vi "自动调阀测试.vi"(8 "error in (no error)":errorcluster caption="错误输入（无错误）") -> (0 "error out":errorcluster caption="错误输出")   [LabVIEW 2015]
doc: "该连续测量范例项目在队列消息处理器模板的基础上实现。\n\n事件处理循环负责按用户界面操作生成对应的消息。\n\n消息处理循环负责对事件处理循环或其他消息生成的消息进行处理。其中还包括用于采集和记录消息处理循环的子VI，以及用于更新图表的循环。"
uses:
  Acquisition/Acquisition.lvlib
  Logging/Logging.lvlib
  support/User Event - Stop/User Event - Stop.lvlib
  support/Message Queue/Message Queue.lvlib
  support/Message Queue/Enqueue Message (Single).vi
  controls/UI Data.ctl
  Measure Type.ctl
  controls/ValueUI Data.ctl
  Action/Action.lvlib
panel:
  out "已完成工序":string
  out "XY Graph":cluster{"Y":dbl[], "Y":dbl[]}[](graph) caption="扭矩VS油压"
  out "XY Graph 2":cluster{"Y":dbl[], "Y":dbl[]}[](graph) caption="角度VS油压"
  out "XY Graph 3":cluster{"Y":dbl[], "Y":dbl[]}[](graph) caption="角度VS扭矩"
  in  "扭杆紧/松":bool
  in  "方向机供油":bool
  in  "夹紧/松阀齿":bool
  in  "夹紧/松阀总":bool
  in  "PLC动作3 5":bool
  in  "PLC动作3 4":bool
  in  "PLC动作3 3":bool
  in  "PLC动作3 2":bool
  in  "PLC动作设置":bool
  in  "PLC动作3":bool
  in  "分中":bool
  in  "转动":bool
  in  "角度":i32
  in  "设置":bool
  in  "清零":bool
  in  "读取":bool
  out "模拟通道5":dbl
  out "流量":dbl
  out "右推力":dbl
  out "左推力":dbl
  out "油压":dbl
  out "扭矩":dbl
  out "角度":dbl
  in  "计算":bool
  in  "Start":bool caption="开始"
  in  "Stop":bool caption="停止"
  out "Status":string caption="状态"
  in  "Exit":bool caption="退出"
  # "力特性测试"
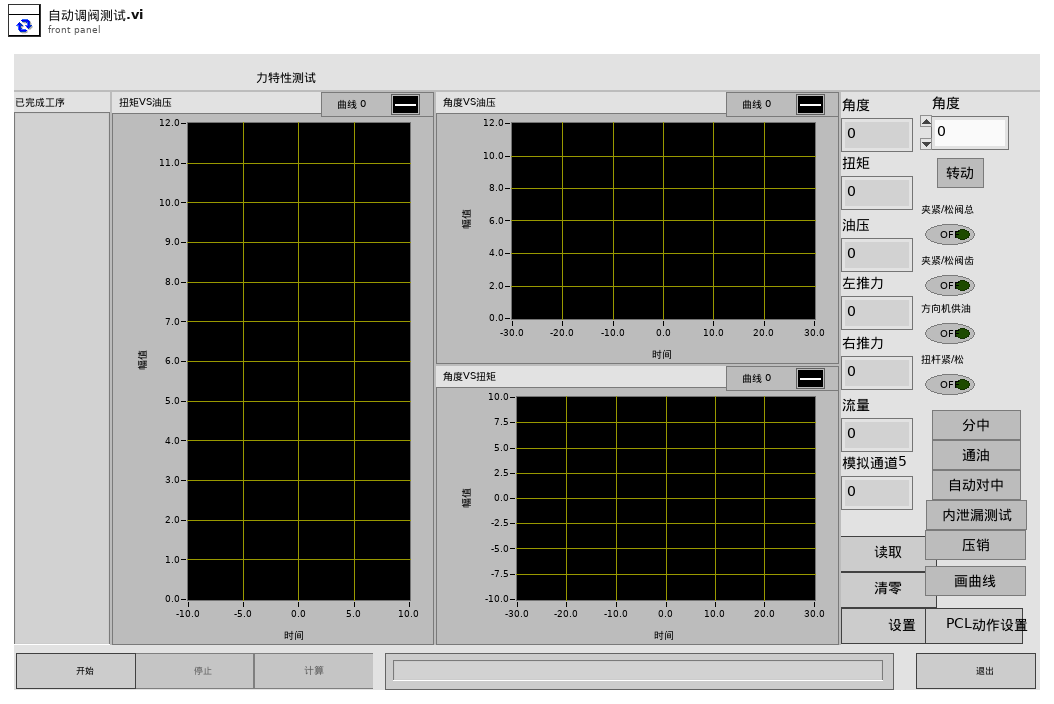
[diagram p1: front panel]
types:
  T1 = typedef "ValueUI Data.ctl" = cluster{"数据1引用":refnum<vi>, "数据2引用":refnum<vi>, "数据3引用":refnum<vi>, "传感器0引用":refnum<vi>, "传感器1引用":refnum<vi>, "传感器2引用":refnum<vi>, "传感器3引用":refnum<vi>, "传感器4引用":refnum<vi>, "传感器5引用":refnum<vi>, "传感器6引用":refnum<vi>}
  T2 = typedef "Measure Type.ctl" = enum16{"啮合", "退回", "功能", "力特性", "内泄漏", "自动调阀测试"}
  T3 = typedef "UI Data.ctl" = cluster{"Start Ref":refnum<vi>, "Stop Ref":refnum<vi>, "calculate Ref":refnum<vi>, "Status Ref":refnum<vi>, "Exit Ref":refnum<vi>, "read Ref":refnum<vi>, "clean Ref":refnum<vi>}
  T4 = typedef "Message Queue.lvlib/All Message Queues.ctl" = cluster{"UI":refnum<queue>, "Acquisition":refnum<queue>, "Logging":refnum<queue>, "plot logic":refnum<queue>, "Action Control":refnum<queue>}
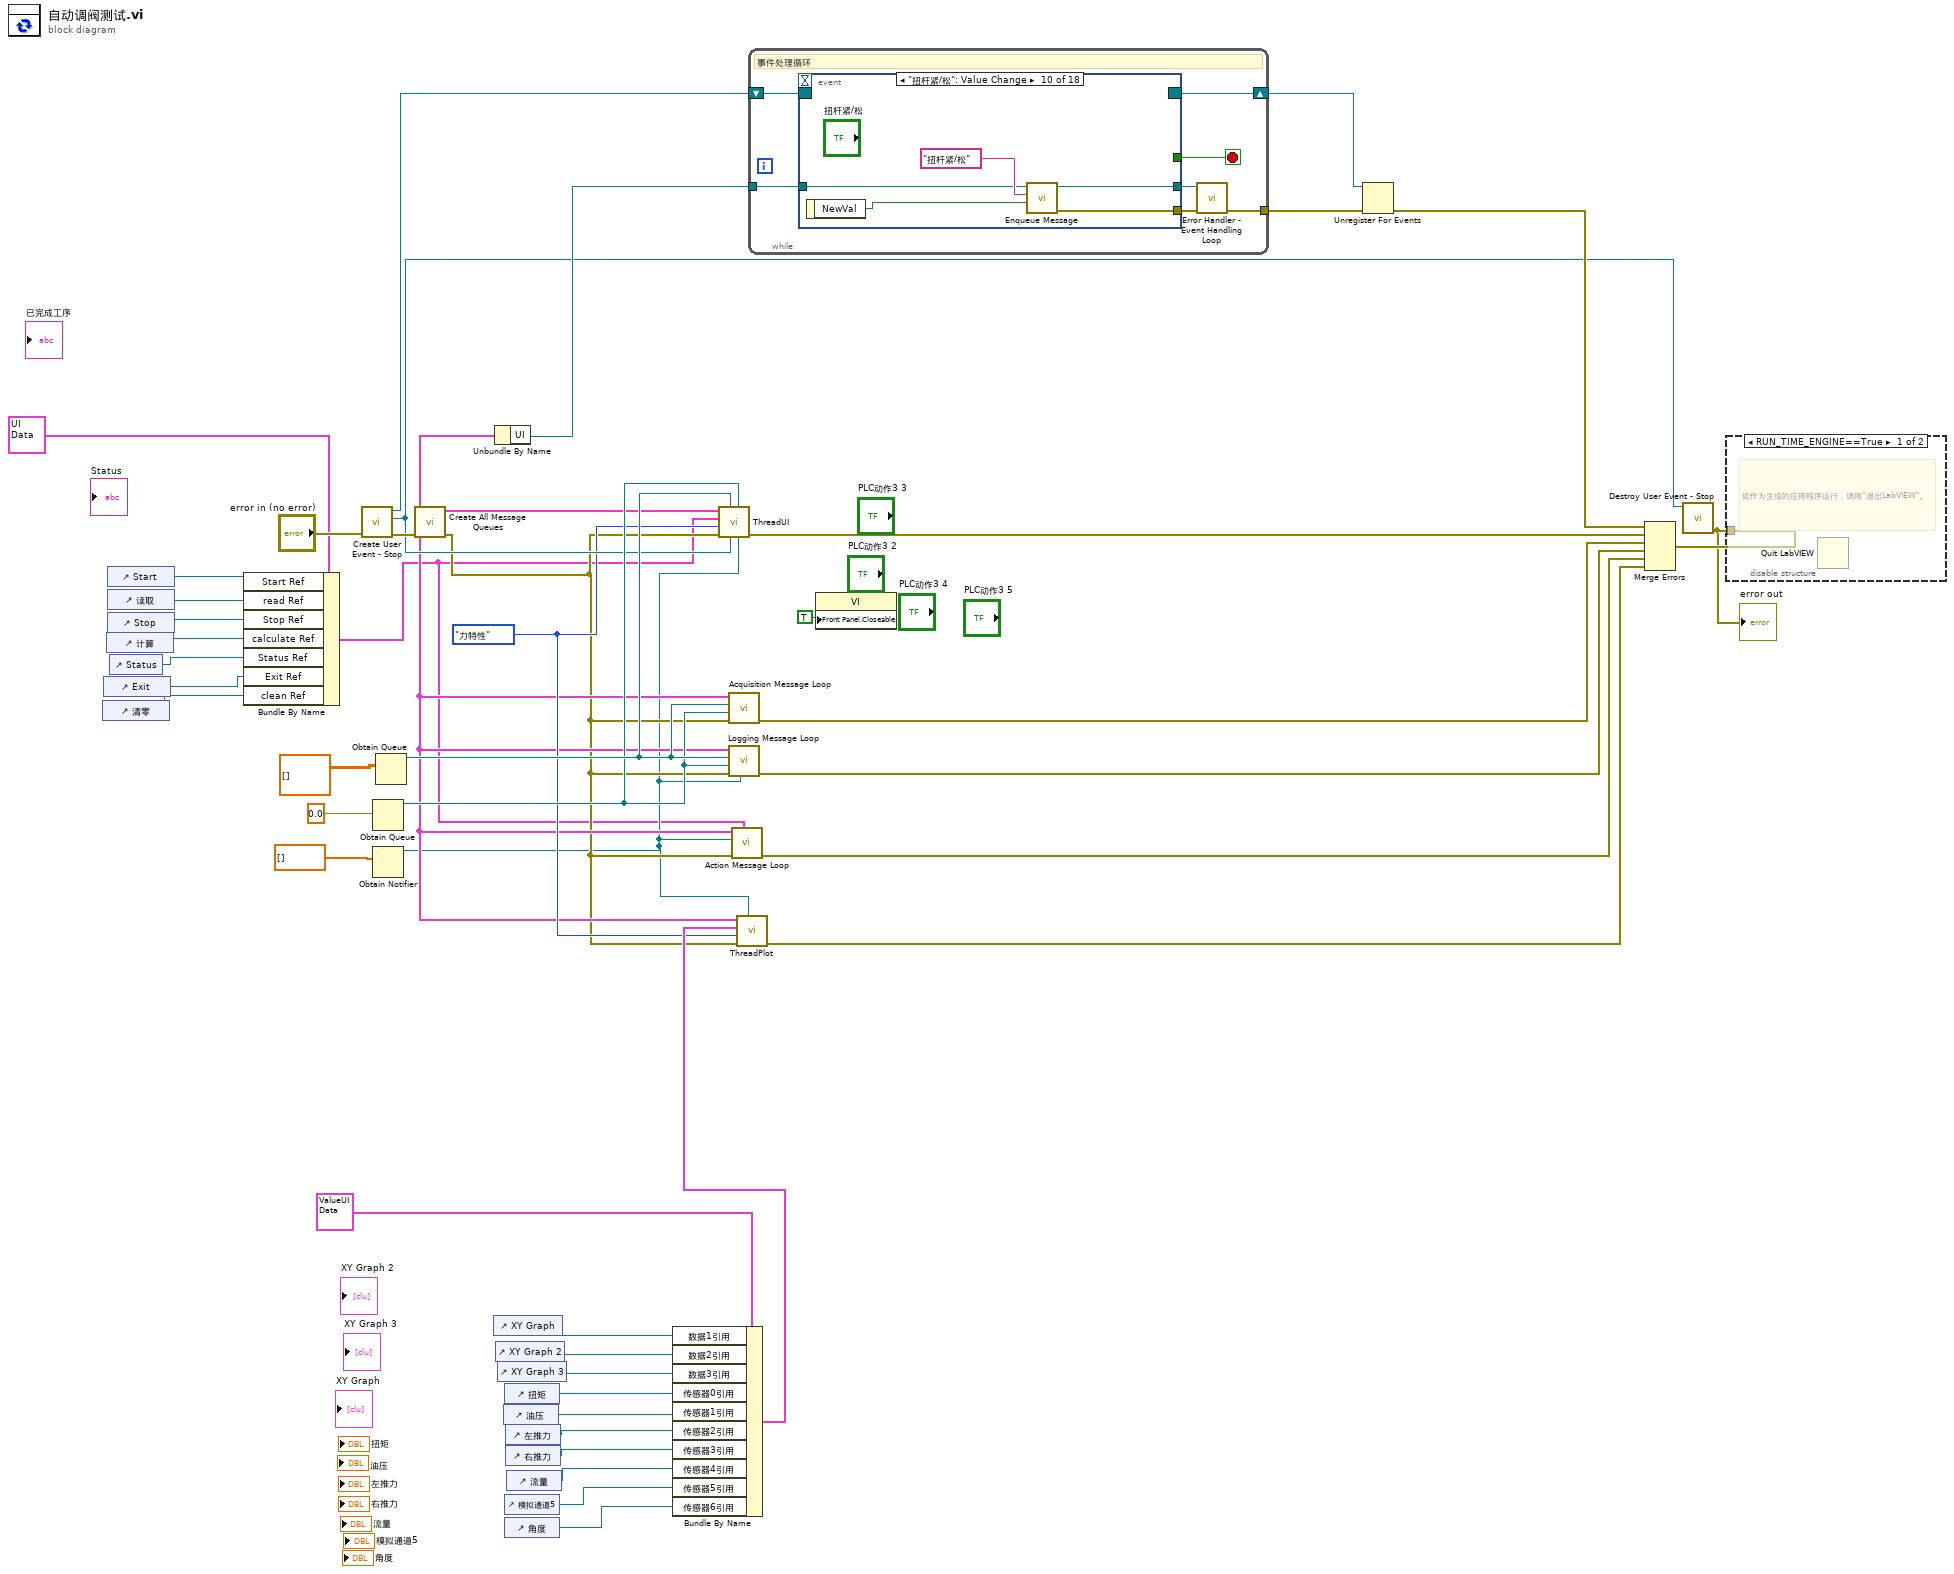
[diagram p0: block diagram]
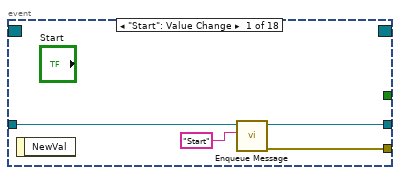
[diagram p3: hidden frame]
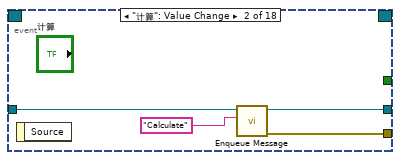
[diagram p4: hidden frame]
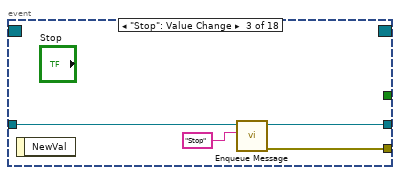
[diagram p5: hidden frame]
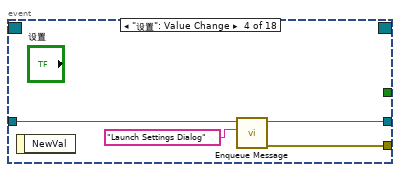
[diagram p6: hidden frame]
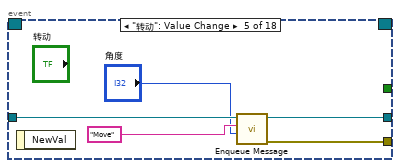
[diagram p7: hidden frame]
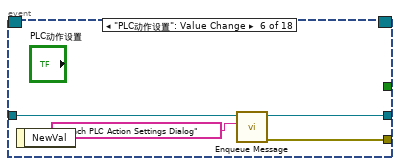
[diagram p8: hidden frame]
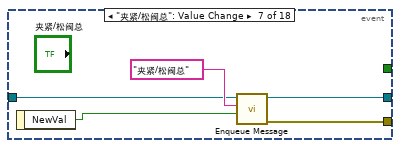
[diagram p9: hidden frame]
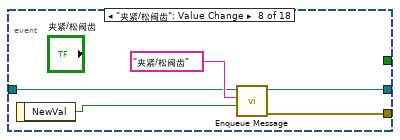
[diagram p10: hidden frame]
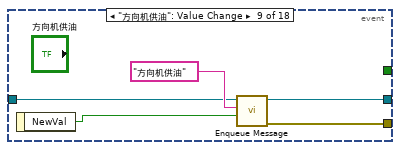
[diagram p11: hidden frame]
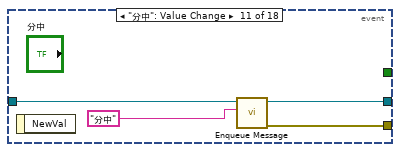
[diagram p12: hidden frame]
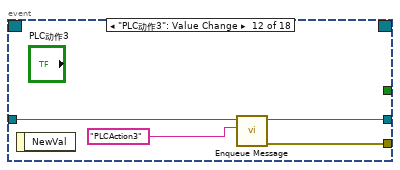
[diagram p13: hidden frame]
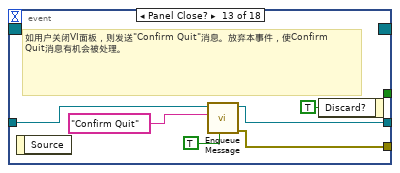
[diagram p14: hidden frame]
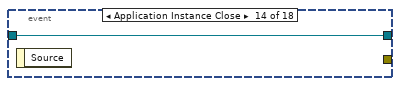
[diagram p15: hidden frame]
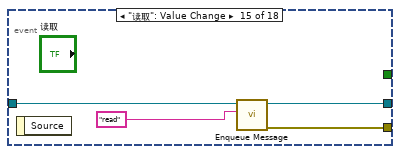
[diagram p16: hidden frame]
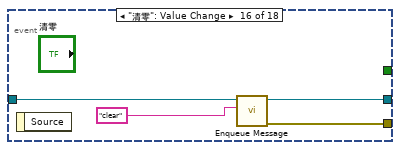
[diagram p17: hidden frame]
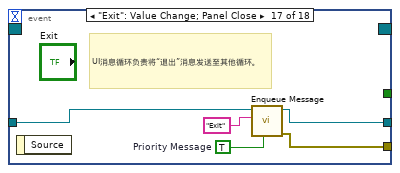
[diagram p18: hidden frame]
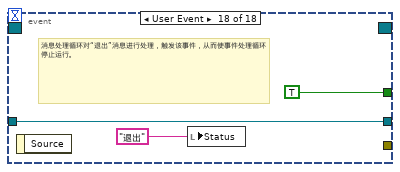
[diagram p19: hidden frame]
diagram:
  w10 = Measure_Type."力特性" ("测试类型")
  n1 = control-ref of="清零"() -> (w26:refnum<vi>)
  n2 = control-ref of="Exit"() -> (w29:refnum<vi>)
  n3 = control-ref of="计算"() -> (w25:refnum<vi>)
  n4 = control-ref of="Start"() -> (w31:refnum<vi>)
  n5 = control-ref of="读取"() -> (w27:refnum<vi>)
  n6 = control-ref of="Stop"() -> (w28:refnum<vi>)
  n7 = control-ref of="Status"() -> (w8:refnum<vi>)
  n8 = Bundle By Name(cluster=T3 {"Start Ref"=refnum, "Stop Ref"=refnum, "calculate Ref"=refnum, "Status Ref"=refnum, "Exit Ref"=refnum, "read Ref"=refnum, "clean Ref"=refnum} ("Measurement UI Controls"), "Start Ref"=w31, "read Ref"=w27, "Stop Ref"=w28, "calculate Ref"=w25, "Status Ref"=w8, "Exit Ref"=w29, "clean Ref"=w26) -> (w1:T3)
  n9 = call "Create User Event - Stop.vi"("error in (no error)"="error in (no error)") -> ("error out"=w42:errorcluster, "User Event - Stop"=w21:refnum<user-event>, "Stop Event Registration Refnum"=w44:refnum<event-registration>)  [unwired: 8 in]
  n10 = Obtain Queue(element data type=0.0) -> (queue out=w23:refnum<queue>)  [unwired: 4 in, 2 out]
  n11 = Obtain Notifier(notification data type=dbl[] []) -> (notifier out=w2:refnum<notifier>)  [unwired: 3 in, 2 out]
  n12 = Obtain Queue(element data type=dbl[][] []) -> (queue out=w24:refnum<queue>)  [unwired: 4 in, 2 out]
  n13 = call "Create All Message Queues.vi"("error in (no error)"=w42) -> ("error out"=w3:errorcluster, "Message Queues out"=w4:T4)  [unwired: 9 in]
  n14 = control-ref of="XY Graph"() -> (w7:refnum<vi>)
  n15 = Unbundle By Name(w4) -> ("UI"=w38:refnum<queue>)
  n16 = control-ref of="XY Graph 2"() -> (w6:refnum<vi>)
  n17 = control-ref of="XY Graph 3"() -> (w5:refnum<vi>)
  n18 = control-ref of="油压"() -> (w17:refnum<vi>)
  n19 = control-ref of="扭矩"() -> (w18:refnum<vi>)
  n20 = control-ref of="模拟通道5"() -> (w13:refnum<vi>)
  n21 = control-ref of="角度"() -> (w12:refnum<vi>)
  n22 = control-ref of="左推力"() -> (w16:refnum<vi>)
  n23 = control-ref of="右推力"() -> (w15:refnum<vi>)
  n24 = control-ref of="流量"() -> (w14:refnum<vi>)
  n25 = Bundle By Name(cluster=T1 {"数据1引用"=refnum, "数据2引用"=refnum, "数据3引用"=refnum, "传感器0引用"=refnum, "传感器1引用"=refnum, "传感器2引用"=refnum, "传感器3引用"=refnum, "传感器4引用"=refnum, "传感器5引用"=refnum, "传感器6引用"=refnum} ("传感器显示UI控件"), "数据1引用"=w7, "数据2引用"=w6, "数据3引用"=w5, "传感器0引用"=w18, "传感器1引用"=w17, "传感器2引用"=w16, "传感器3引用"=w15, "传感器4引用"=w14, "传感器5引用"=w13, "传感器6引用"=w12) -> (w11:T1)
  n26 = call "ThreadUI.vi"("数据通知器"=w2, "Angle Data Queue"=w23, "User Event - Stop"=w21, "Analog Data Queue"=w24, "error in (no error)"=w3, "测试类型"=w10, "Measurement UI Controls"=w1, "Message Queues"=w4) -> ("error out"=w20:errorcluster)  [unwired: 3 in]
  n27 = call "Acquisition Message Loop.vi"("error in (no error)"=w3, "Angle Data Queue"=w23, "Analog Data Queue"=w24, "Message Queues"=w4) -> ("error out"=w43:errorcluster)  [unwired: 7 in]
  n28 = call "Logging Message Loop.vi"("数据通知器"=w2, "error in (no error)"=w3, "Angle Data Queue"=w23, "Analog Data Queue"=w24, "Message Queues"=w4) -> ("error out"=w41:errorcluster)  [unwired: 6 in]
  n29 = call "Action Message Loop.vi"("Measurement UI Controls"=w1, "error in (no error)"=w3, "Data Notifier"=w2, "Message Queues"=w4) -> ("error out"=w34:errorcluster)  [unwired: 7 in]
  n30 = call "ThreadPlot.vi"("数据通知器"=w2, "error in (no error)"=w3, "测试类型"=w10, "传感器显示UI控件"=w11, "Message Queues"=w4) -> ("error out"=w9:errorcluster)  [unwired: 6 in]
  n31 = while {
    tunnel: w38 -> [w52]
    tunnel: [w47] -> w46
    shift-right: [w51] -> w39
    shift-left: w44 -> [w53]
    stop <- w50 stop-if-true
    # "事件处理循环"
    n32 = event shown="[9] \"扭杆紧/松\": Value Change" {
      selector: w53 -> [_ _ _ _ _ _ _ _ _ _ _ _ _ _ _ _ _ _]
      dyn-events: [_ _ _ _ _ _ _ _ _ _ _ _ _ _ _ _ _ _] -> w51
      timeout: _ -> [_ _ _ _ _ _ _ _ _ _ _ _ _ _ _ _ _ _]
      tunnel: [_ _ _ _ _ _ _ _ _ _ _ _ _ _ _ _ _ TRUE ("Discard?")] -> w50
      tunnel: w52 -> [w55 w60 w64 w68 w73 w77 w82 w87 w92 w97 w101 w105 w112 w113 w115 w119 w123 w127]
      tunnel: [w57 w59 w63 w67 w72 w76 w81 w86 w91 w96 w100 w104 w107 _ w117 w121 w126 _] -> w48
      tunnel: [w54 w58 w62 w66 w71 w75 w80 w85 w90 w95 w99 w103 w108 w113 w114 w118 w122 w127] -> w49
      event "Start": Value Change {
        n33 = event-data() -> ()  [unwired: 1 in, 1 out]
        n34 = call-poly "Enqueue Message.vi"("Message"="Start", "Message Queue"=w55) -> ("error out"=w57:errorcluster, "dup Message Queue"=w54:refnum<queue>)  [unwired: 8 in]
      }
      event "计算": Value Change {
        n35 = event-data() -> ()  [unwired: 1 in, 1 out]
        n36 = call-poly "Enqueue Message.vi"("Message"="Calculate", "Message Queue"=w60) -> ("error out"=w59:errorcluster, "dup Message Queue"=w58:refnum<queue>)  [unwired: 8 in]
      }
      event "Stop": Value Change {
        n37 = event-data() -> ()  [unwired: 1 in, 1 out]
        n38 = call-poly "Enqueue Message.vi"("Message"="Stop", "Message Queue"=w64) -> ("error out"=w63:errorcluster, "dup Message Queue"=w62:refnum<queue>)  [unwired: 8 in]
      }
      event "设置": Value Change {
        n39 = event-data() -> ()  [unwired: 1 in, 1 out]
        n40 = call-poly "Enqueue Message.vi"("Message"="Launch Settings Dialog", "Message Queue"=w68) -> ("error out"=w67:errorcluster, "dup Message Queue"=w66:refnum<queue>)  [unwired: 8 in]
      }
      event "转动": Value Change {
        n41 = event-data() -> ()  [unwired: 1 in, 1 out]
        n42 = call-poly "Enqueue Message.vi"("Message Data"="角度", "Message"="Move", "Message Queue"=w73) -> ("error out"=w72:errorcluster, "dup Message Queue"=w71:refnum<queue>)  [unwired: 7 in]
      }
      event "PLC动作设置": Value Change {
        n43 = event-data() -> ()  [unwired: 1 in, 1 out]
        n44 = call-poly "Enqueue Message.vi"("Message"="Launch PLC Action Settings Dialog", "Message Queue"=w77) -> ("error out"=w76:errorcluster, "dup Message Queue"=w75:refnum<queue>)  [unwired: 8 in]
      }
      event "夹紧/松阀总": Value Change {
        n45 = event-data() -> ("NewVal"=w79:bool)  [unwired: 1 in]
        n46 = call-poly "Enqueue Message.vi"("Message Data"=w79, "Message"="夹紧/松阀总", "Message Queue"=w82) -> ("error out"=w81:errorcluster, "dup Message Queue"=w80:refnum<queue>)  [unwired: 7 in]
      }
      event "夹紧/松阀齿": Value Change {
        n47 = event-data() -> ("NewVal"=w84:bool)  [unwired: 1 in]
        n48 = call-poly "Enqueue Message.vi"("Message Data"=w84, "Message"="夹紧/松阀齿", "Message Queue"=w87) -> ("error out"=w86:errorcluster, "dup Message Queue"=w85:refnum<queue>)  [unwired: 7 in]
      }
      event "方向机供油": Value Change {
        n49 = event-data() -> ("NewVal"=w89:bool)  [unwired: 1 in]
        n50 = call-poly "Enqueue Message.vi"("Message Data"=w89, "Message"="方向机供油", "Message Queue"=w92) -> ("error out"=w91:errorcluster, "dup Message Queue"=w90:refnum<queue>)  [unwired: 7 in]
      }
      event "扭杆紧/松": Value Change {
        n51 = event-data() -> ("NewVal"=w94:bool)  [unwired: 1 in]
        n52 = call-poly "Enqueue Message.vi"("Message Data"=w94, "Message"="扭杆紧/松", "Message Queue"=w97) -> ("error out"=w96:errorcluster, "dup Message Queue"=w95:refnum<queue>)  [unwired: 7 in]
      }
      event "分中": Value Change {
        n53 = event-data() -> ()  [unwired: 1 in, 1 out]
        n54 = call-poly "Enqueue Message.vi"("Message"="分中", "Message Queue"=w101) -> ("error out"=w100:errorcluster, "dup Message Queue"=w99:refnum<queue>)  [unwired: 8 in]
      }
      event "PLC动作3": Value Change {
        n55 = event-data() -> ()  [unwired: 1 in, 1 out]
        n56 = call-poly "Enqueue Message.vi"("Message"="PLCAction3", "Message Queue"=w105) -> ("error out"=w104:errorcluster, "dup Message Queue"=w103:refnum<queue>)  [unwired: 8 in]
      }
      event Panel Close? {
        # "如用户关闭VI面板，则发送\"Confirm Quit\"消息。放弃本事件，使Confirm Quit消息有机会被处理。"
        n57 = event-data() -> ()  [unwired: 1 in, 1 out]
        n58 = call-poly "Enqueue Message.vi"("Priority Message? (F)"=TRUE, "Message"="Confirm Quit", "Message Queue"=w112) -> ("error out"=w107:errorcluster, "dup Message Queue"=w108:refnum<queue>)  [unwired: 7 in]
        n59 = event-data("Discard?"=TRUE) -> ()  [unwired: 1 in, 1 out]
      }
      event Application Instance Close {
        n60 = event-data() -> ()  [unwired: 1 in, 1 out]
      }
      event "读取": Value Change {
        n61 = event-data() -> ()  [unwired: 1 in, 1 out]
        n62 = call-poly "Enqueue Message.vi"("Message"="read", "Message Queue"=w115) -> ("error out"=w117:errorcluster, "dup Message Queue"=w114:refnum<queue>)  [unwired: 8 in]
      }
      event "清零": Value Change {
        n63 = event-data() -> ()  [unwired: 1 in, 1 out]
        n64 = call-poly "Enqueue Message.vi"("Message"="clear", "Message Queue"=w119) -> ("error out"=w121:errorcluster, "dup Message Queue"=w118:refnum<queue>)  [unwired: 8 in]
      }
      event "Exit": Value Change; Panel Close {
        w124 = TRUE  # Priority Message
        # "UI消息循环负责将“退出”消息发送至其他循环。"
        n65 = event-data() -> ()  [unwired: 1 in, 1 out]
        n66 = call-poly "Enqueue Message.vi"("Priority Message? (F)"=w124, "Message"="Exit", "Message Queue"=w123) -> ("error out"=w126:errorcluster, "dup Message Queue"=w122:refnum<queue>)  [unwired: 7 in]
      }
      event User Event {
        # "消息处理循环对“退出”消息进行处理，触发该事件，从而使事件处理循环停止运行。"
        n67 = event-data() -> ()  [unwired: 1 in, 1 out]
        n68 = local write "Status"("退出" ("Exit String")) -> ()
      }
    }
    n69 = call "Error Handler - Event Handling Loop.vi"("error in (no error)"=w48, "Message Queue"=w49) -> ("dup error in"=w47:errorcluster)  [unwired: 8 in, 1 out]
  }
  n70 = property class="VI"("Front Panel.Closeable"=TRUE ("Front Panel Window:Closeable")) -> ()  [unwired: 2 in, 2 out]
  n71 = Unregister For Events(event registration refnum=w39, error in=w46) -> (error out=w40:errorcluster)
  n72 = Merge Errors(w40, w20, w43, w41, w34, w9) -> (w45:errorcluster)
  n73 = call "Destroy User Event - Stop.vi"("error in (no error)"=w45, "User Event - Stop"=w21) -> ("error out"=w33:errorcluster)  [unwired: 9 in]
  "error out" <- w33
  n74 = disable-structure shown="RUN_TIME_ENGINE==True" {
    disable-tunnel: w33 -> [_ _]
    frame condition #0 {
      # "如作为生成的应用程序运行，调用“退出LabVIEW”。"
      n75 = Quit LabVIEW() -> ()  [unwired: 1 in]
    }
    frame condition #1 (active) {
    }
  }
